vi "Thread@SubThreadEnd__Parameter.vi"(1 "ParamterIn":string) -> (0 "ParamterOut":string)   [LabVIEW 2020]
uses:
  MainFrame/Global.vi
panel:
  in  "Thread Label":string(combo)
  in  "Confirm":bool
  # "Thread@SubThreadEnd $SubName"
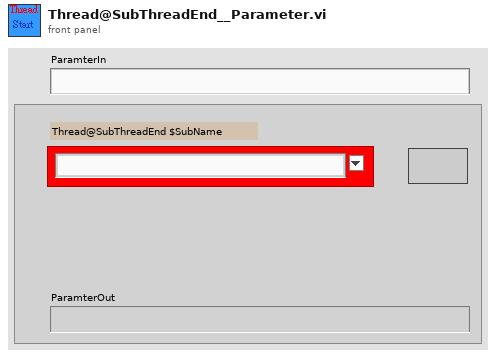
[diagram p1: front panel]
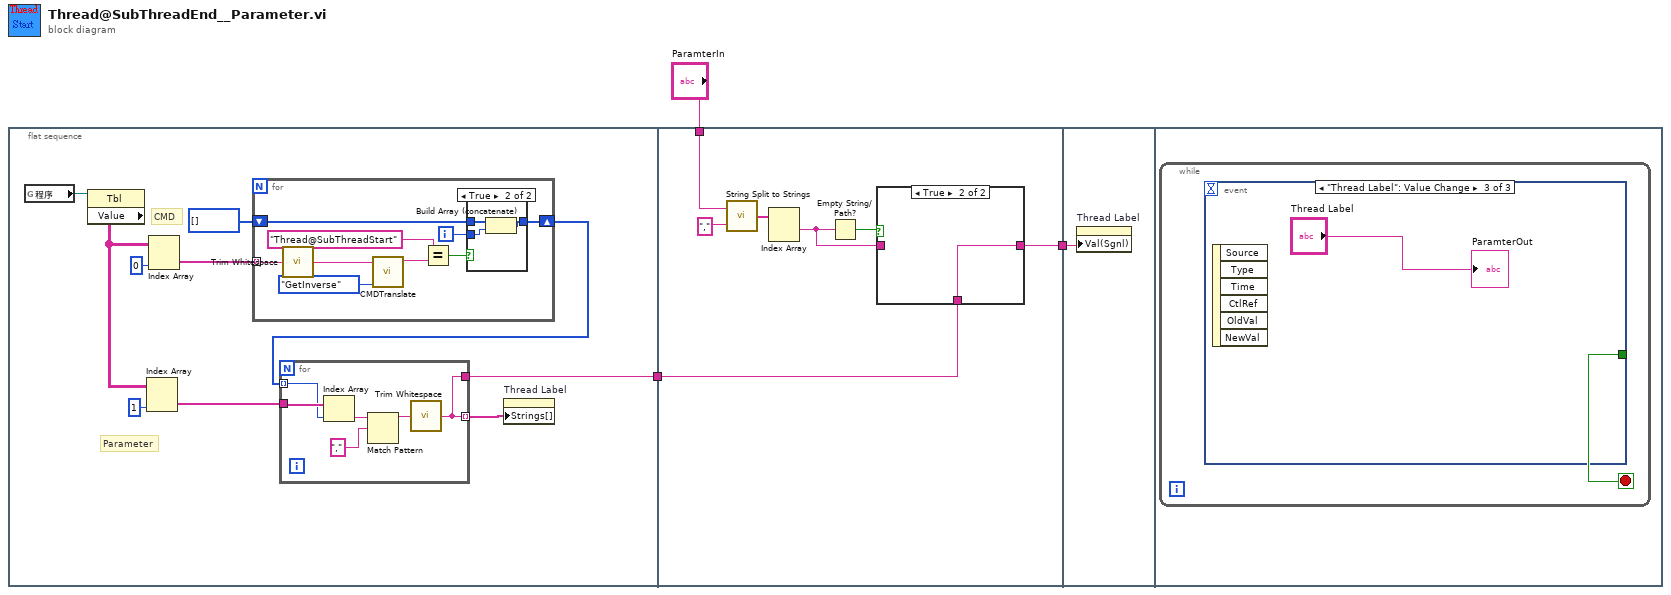
[diagram p0: block diagram]
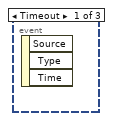
[diagram p4: hidden frame]
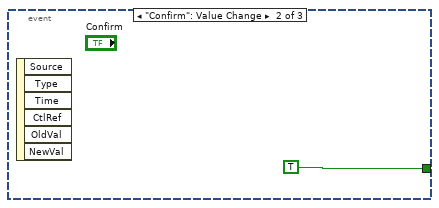
[diagram p5: hidden frame]
diagram:
  n1 = flat-sequence {
    tunnel: [w4] -> w1
    tunnel: "ParamterIn" -> [w37]
    tunnel: [w34] -> w2
    tunnel: w1 -> [w33]
    tunnel: w2 -> [w42]
    frame #0 {
      # "Parameter"
      # "CMD"
      n2 = global read "Global.vi" "程序"() -> (w13:refnum<vi>)
      n3 = property class="Tbl"(reference=w13) -> ("Value"=w10:string[][])  [unwired: 1 in, 2 out]
      n4 = Index Array(array=w10, index (col)=1 ("index (row)")) -> (element=w7:string[])  [unwired: 1 in]
      n5 = Index Array(array=w10, index (col)=0 ("index (row)")) -> (element=w9:string[])  [unwired: 1 in]
      n6 = for {
        tunnel: w9 -> [w21] mode=indexing
        shift-right: [w22] -> w6
        shift-left: i32[] [] -> [w24]
        i -> [w23]
        n7 = call <vilib>:"Trim Whitespace.vi"("string"=w21) -> ("trimmed string"=w20:string)  [unwired: 1 in]
        n8 = call "CMDTranslate.vi"("OP"=enum16{"Init", "Set", "Get", "GetInverse"}."GetInverse", "CMDIn"=w20) -> ("CMDOut"=w27:string)  [unwired: 9 in]
        n9 = Equal?(x="Thread@SubThreadStart", y=w27) -> (x = y?=w25:bool)
        n10 = case shown="True" w25 {
          tunnel: w24 -> [w29 w32]
          tunnel: w23 -> [_ w31]
          tunnel: [w29 w30] -> w22
          frame False {
          }
          frame True {
            n11 = Build Array (concatenate)(w32, w31) -> (w30:i32[])
          }
        }
      }
      n12 = for {
        tunnel: w7 -> [w19]
        tunnel: w6 -> [w18] mode=indexing
        tunnel: [w15] -> w5 mode=indexing
        tunnel: [w15] -> w4
        n13 = Index Array(array=w19, index=w18) -> (element=w17:string)
        n14 = Match Pattern(string=w17, regular expression=",") -> (before substring=w14:string)  [unwired: 1 in, 3 out]
        n15 = call <vilib>:"Trim Whitespace.vi"("string"=w14) -> ("trimmed string"=w15:string)  [unwired: 1 in]
      }
      n16 = property on="Thread Label" class="CmbBox"("Strings[]"=w5) -> ()  [unwired: 2 in, 2 out]
    }
    frame #1 {
      n17 = call "String Split to Strings.vi"("search string/char (-)"=",", "String"=w37) -> ("Array"=w39:string[])
      n18 = Index Array(array=w39) -> (element #1=w35:string)  [unwired: 2 in, 1 out]
      n19 = Empty String/Path?(string/path=w35) -> (empty?=w36:bool)
      n20 = case shown="True" w36 {
        tunnel: w35 -> [w40 _]
        tunnel: [w40 w41] -> w34
        tunnel: w33 -> [_ w41]
        frame False {
        }
        frame True {
        }
      }
    }
    frame #2 {
      n21 = property on="Thread Label" class="CmbBox"("Val(Sgnl)"=w42) -> ()  [unwired: 2 in, 2 out]
    }
    frame #3 {
      n22 = while {
        stop <- w43 stop-if-true
        n23 = event shown="[2] \"Thread Label\": Value Change" {
          selector: _ -> [_ _ _]
          dyn-events: _ -> [_ _ _]
          timeout: _ -> [_ _ _]
          tunnel: [_ TRUE _] -> w43
          event Timeout {
            n24 = event-data() -> ()  [unwired: 1 in, 3 out]
          }
          event "Confirm": Value Change {
            n25 = event-data() -> ()  [unwired: 1 in, 6 out]
          }
          event "Thread Label": Value Change {
            n26 = event-data() -> ()  [unwired: 1 in, 6 out]
            "ParamterOut" <- "Thread Label"
          }
        }
      }
    }
  }
